vi "Diagnostic Sample.vi"(8 "error in (no error)":errorcluster, 10 "Acquisition Data":T1, 11 "CAP-USB-1 in":refnum<class "CAP-USB-1.lvclass">) -> (0 "error out":errorcluster, 2 "Acquisition Data":T1, 3 "CAP-USB-1 out":refnum<class "CAP-USB-1.lvclass">)   [LabVIEW 2014, in "CAP-USB-1.lvlib" / "CAP-USB-1.lvclass"]
doc: "Verifica que el valor de cada muestra este dentro de los parametros configurados"
uses:
  CAP-USB-1.lvclass
  DriverMasterSync/build/DriverMasterSync.lvlibp/APIs/Data Queue/Acquisition Data Cluster.ctl
  DriverMasterSync/build/DriverMasterSync.lvlibp/APIs/Data Queue/Acquisition Data 1 Sample Cluster.ctl
  CAP-USB-1.lvclass/CAP-USB-1.ctl
  DriverMasterSync/build/DriverMasterSync.lvlibp/APIs/Data Queue/WINFAS 2 Data Queue.lvlib
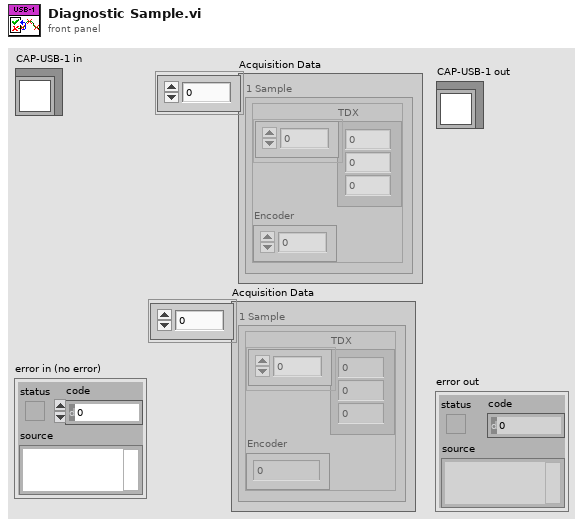
[diagram p1: front panel]
types:
  T1 = typedef "DriverMasterSync.lvlibp/WINFAS 2 Data Queue.lvlib/Acquisition Data Cluster.ctl" = T2[]
  T2 = typedef "DriverMasterSync.lvlibp/WINFAS 2 Data Queue.lvlib/Acquisition Data 1 Sample Cluster.ctl" = cluster{"TDX":sgl[], "Encoder":sgl}
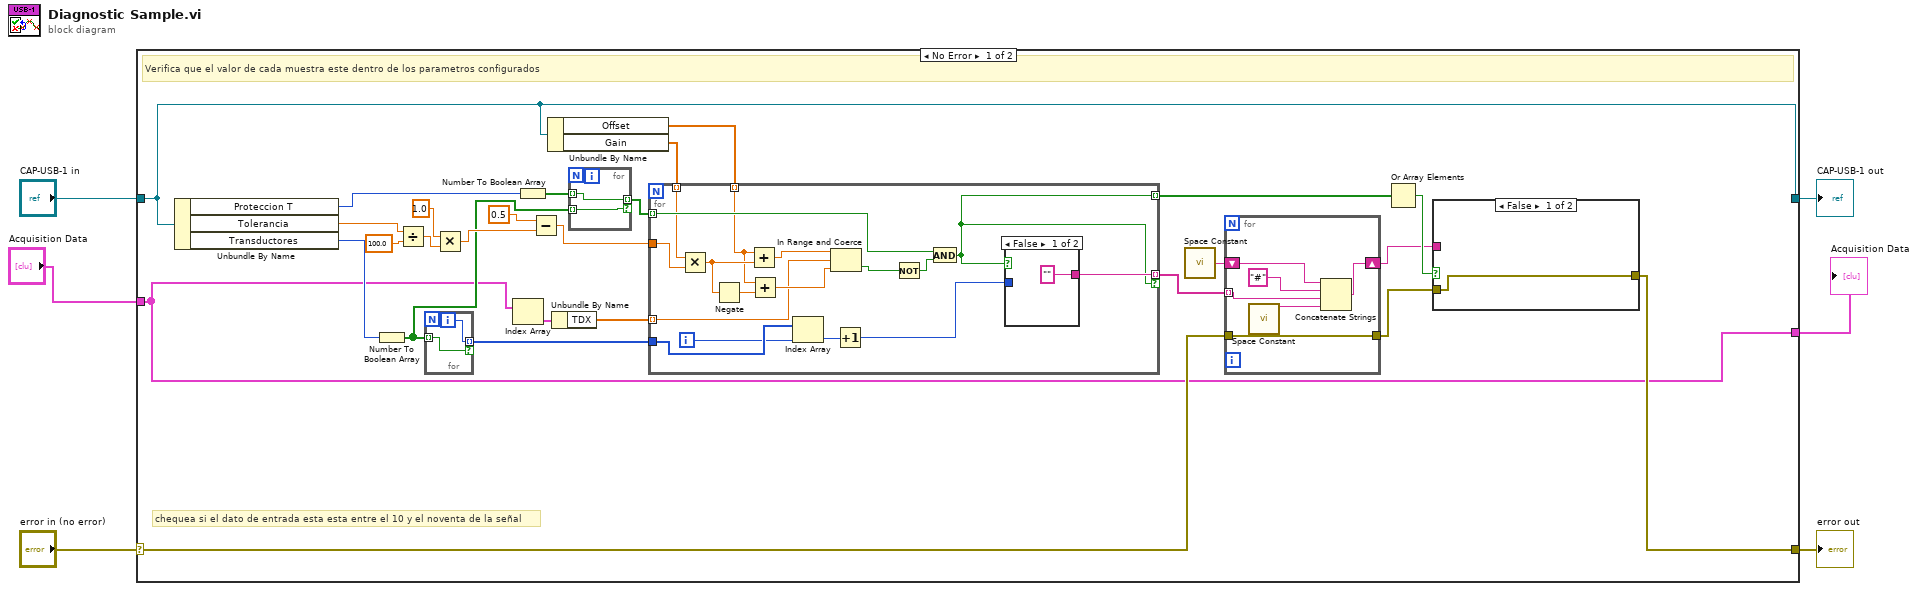
[diagram p0: block diagram]
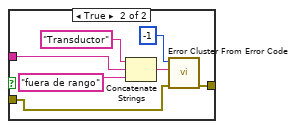
[diagram p2: hidden frame]
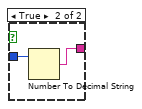
[diagram p3: hidden frame]
diagram:
  n1 = case shown="No Error" "error in (no error)" {
    selector: "error in (no error)" -> [w20 w74]
    tunnel: [w27 w74] -> w5
    tunnel: [w9 w73] -> w3
    tunnel: "CAP-USB-1 in" -> [w9 w73]
    tunnel: "Acquisition Data" -> [w12 w72]
    tunnel: [w12 w72] -> w1
    frame No Error {
      # "chequea si el dato de entrada esta esta entre el 10 y el noventa de la señal"
      # "Verifica que el valor de cada muestra este dentro de los parametros configurados"
      n2 = Unbundle By Name(w9) -> ("Proteccion T"=w23:u64, "Tolerancia"=w33:sgl, "Transductores"=w26:u64)
      n3 = Number To Boolean Array(number=w26) -> (Boolean array=w13:bool[])
      n4 = Divide(x=w33, y=sgl 100.0) -> (x/y=w31:sgl)
      n5 = for {
        tunnel: w13 -> [w50] mode=indexing
        tunnel: [w51] -> w25 mode=indexing if=w50
        i -> [w51]
      }
      n6 = Multiply(x=sgl 1.0, y=w31) -> (x*y=w30:sgl)
      n7 = Index Array(array=w12) -> (element=w11:T2)  [unwired: 1 in]
      n8 = Number To Boolean Array(number=w23) -> (Boolean array=w15:bool[])
      n9 = Subtract(x=sgl 0.5, y=w30) -> (x-y=w28:sgl)
      n10 = Unbundle By Name(w9) -> ("Offset"=w8:sgl[], "Gain"=w7:sgl[])
      n11 = Unbundle By Name(w11) -> ("TDX"=w10:sgl[])
      n12 = for {
        tunnel: w15 -> [w35] mode=indexing
        tunnel: [w35] -> w14 mode=indexing if=w34
        tunnel: w13 -> [w34] mode=indexing
      }
      n13 = for {
        tunnel: w28 -> [w58]
        tunnel: w25 -> [w67]
        tunnel: w14 -> [w68] mode=indexing
        tunnel: [w62] -> w22 mode=indexing
        tunnel: [w63] -> w17 mode=indexing if=w62
        tunnel: w10 -> [w52] mode=indexing
        tunnel: w8 -> [w56] mode=indexing
        tunnel: w7 -> [w59] mode=indexing
        i -> [w66]
        n14 = Multiply(x=w59, y=w58) -> (x*y=w57:sgl)
        n15 = Negate(x=w57) -> (-x=w55:sgl)
        n16 = Add(x=w56, y=w57) -> (x+y=w54:sgl)
        n17 = Add(x=w56, y=w55) -> (x+y=w53:sgl)
        n18 = Index Array(array=w67, index=w66) -> (element=w65:i32)
        n19 = In Range and Coerce(upper limit=w54, x=w52, lower limit=w53) -> (In Range?=w61:bool)  [unwired: 1 out]
        n20 = Increment(x=w65) -> (x+1=w64:i32)
        n21 = Not(x=w61) -> (.not. x?=w60:bool)
        n22 = And(x=w68, y=w60) -> (x .and. y?=w62:bool)
        n23 = case shown="False" w62 {
          tunnel: ["" w71] -> w63
          tunnel: w64 -> [_ w70]
          frame False {
          }
          frame True {
            n24 = Number To Decimal String(number=w70) -> (decimal integer string=w71:string)  [unwired: 1 in]
          }
        }
      }
      n25 = call <vilib>:"Space Constant.vi"() -> ("String"=w16:string)
      n26 = for {
        tunnel: [w41] -> w19
        tunnel: w20 -> [w41]
        shift-right: [w40] -> w18
        shift-left: w16 -> [w39]
        tunnel: w17 -> [w36] mode=indexing
        n27 = call <vilib>:"Space Constant.vi"() -> ("String"=w37:string)
        n28 = Concatenate Strings(w39, "#" ("string"), w36, w37) -> (w40:string)
      }
      n29 = Or Array Elements(Boolean array=w22) -> (logical OR=w21:bool)
      n30 = case shown="False" w21 {
        tunnel: [w42 w49] -> w27
        tunnel: w19 -> [w42 w44]
        tunnel: w18 -> [_ w43]
        frame False {
        }
        frame True {
          n31 = Concatenate Strings("Transductor", w43, "fuera de rango" ("string")) -> (w46:string)
          n32 = call <vilib>:"Error Cluster From Error Code.vi"("error in (no error)"=w44, "error message (\"\")"=w46, "error code (0)"=-1) -> ("error out"=w49:errorcluster)  [unwired: 6 in]
        }
      }
    }
    frame Error {
    }
  }
  "error out" <- w5
  "CAP-USB-1 out" <- w3
  "Acquisition Data" <- w1
